vi "Side Motion Calculator.vi"(8 "Error In":errorcluster, 10 "Numeric 2":dbl, 11 "Numeric":dbl) -> (0 "Error out":errorcluster, 3 "Numeric 3":dbl)   [LabVIEW 2018]
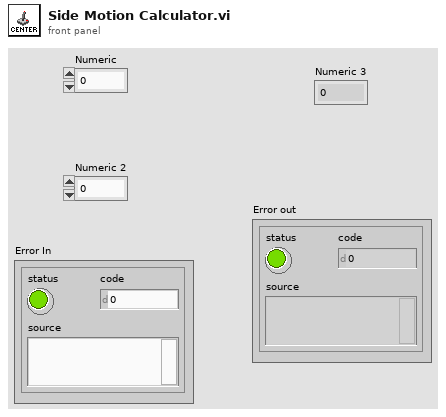
[diagram p1: front panel]
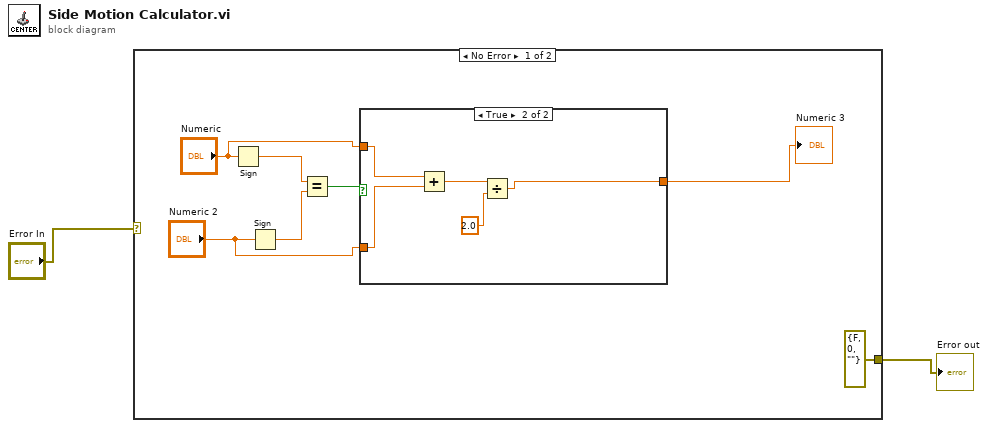
[diagram p0: block diagram]
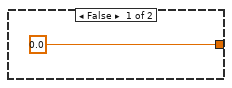
[diagram p2: hidden frame]
diagram:
  n1 = case shown="No Error" "Error In" {
    selector: "Error In" -> [_ w16]
    tunnel: [errorcluster {"status"=FALSE, "code"=0, "source"=""} ("error IO") w16] -> w1
    frame No Error {
      n2 = Sign(1:"Numeric") -> (0:w9:dbl)
      n3 = Sign(1:"Numeric 2") -> (0:w8:dbl)
      n4 = Equal?(x=w9, y=w8) -> (x = y?=w7:bool)
      n5 = case shown="True" w7 {
        tunnel: [0.0 w11] -> w6
        tunnel: "Numeric" -> [_ w15]
        tunnel: "Numeric 2" -> [_ w14]
        frame False {
        }
        frame True {
          n6 = Add(x=w15, y=w14) -> (x+y=w12:dbl)
          n7 = Divide(x=w12, y=2.0) -> (x/y=w11:dbl)
        }
      }
      "Numeric 3" <- w6
    }
    frame Error {
    }
  }
  "Error out" <- w1
